vi "reset_TRIG2.vi"(8 "error in (no error)":errorcluster, 11 "VISA resource name":refnum<visa-resource-name>) -> (0 "error out":errorcluster, 3 "VISA resource name out":refnum<visa-resource-name>)   [LabVIEW 2011]
doc: "This vi resets TRIG2 (DG645) to its defaultsetup and then configures a default setup for the chirped pulse setup.\nThis includes activating the burst mode (3 bursts, 100us burst period), setting polarities as well as setting all delays and durations to 0."
uses:
  global.vi
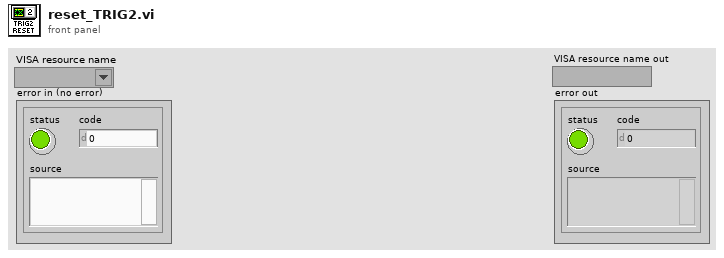
[diagram p1: front panel]
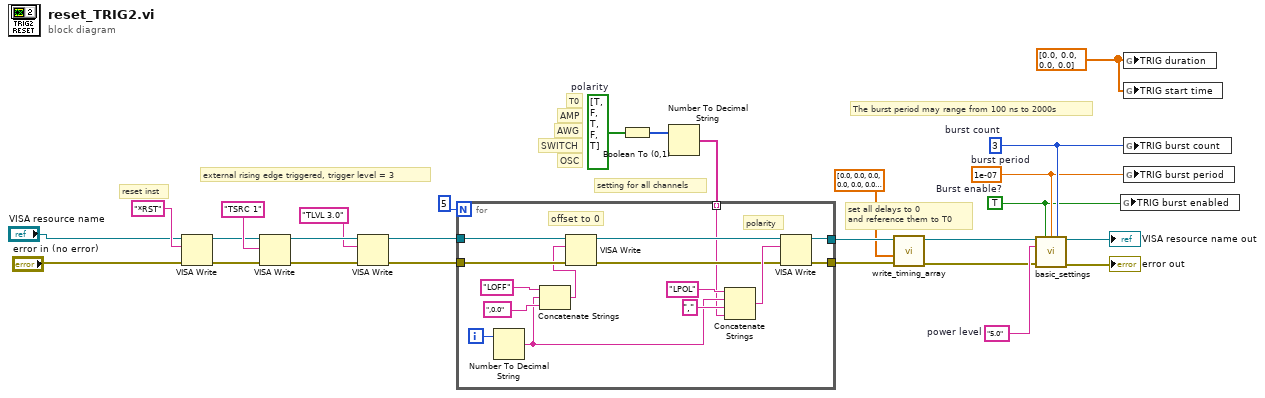
[diagram p0: block diagram]
diagram:
  w6 = bool[] [TRUE, FALSE, TRUE, FALSE, TRUE]  # polarity
  w9 = dbl[] [0.0, 0.0, 0.0, 0.0] ("duration")
  w16 = 3  # burst count
  w15 = 1e-07  # burst period
  w14 = TRUE  # Burst enable?
  w21 = "5.0"  # power level
  # "OSC"
  # "SWITCH"
  # "AWG"
  # "AMP"
  # "T0"
  # "The burst period may range from 100 ns to 2000s"
  # "set all delays to 0 \nand reference them to T0"
  # "reset inst"
  # "setting for all channels"
  # "external rising edge triggered, trigger level = 3"
  n1 = VISA Write(VISA resource name="VISA resource name", write buffer="*RST", error in (no error)="error in (no error)") -> (VISA resource name out=w23:refnum<visa-resource-name>, error out=w24:errorcluster)  [unwired: 1 out]
  n2 = VISA Write(VISA resource name=w23, write buffer="TSRC 1" ("Query 2"), error in (no error)=w24) -> (VISA resource name out=w3:refnum<visa-resource-name>, error out=w25:errorcluster)  [unwired: 1 out]
  n3 = VISA Write(VISA resource name=w3, write buffer="TLVL 3.0", error in (no error)=w25) -> (VISA resource name out=w2:refnum<visa-resource-name>, error out=w4:errorcluster)  [unwired: 1 out]
  n4 = Boolean To (0,1)(Boolean=w6) -> (0, 1=w7:i16[])
  n5 = Number To Decimal String(number=w7) -> (decimal integer string=w5:string[])  [unwired: 1 in]
  n6 = for {
    N: 5 -> [_]
    tunnel: w2 -> [w40]
    tunnel: [w31] -> w13
    tunnel: w4 -> [w39]
    tunnel: [w30] -> w12
    tunnel: w5 -> [w28] mode=indexing
    i -> [w38]
    # "polarity"
    # "offset to 0"
    n7 = Number To Decimal String(number=w38) -> (decimal integer string=w29:string)  [unwired: 1 in]
    n8 = Concatenate Strings("LOFF" ("Query 2"), w29, ",0.0" ("Query 2")) -> (w35:string)
    n9 = VISA Write(VISA resource name=w40, write buffer=w35, error in (no error)=w39) -> (VISA resource name out=w31:refnum<visa-resource-name>, error out=w30:errorcluster)  [unwired: 1 out]
    n10 = Concatenate Strings("LPOL" ("Query 2"), w29, "," ("string"), w28) -> (w33:string)
    n11 = VISA Write(VISA resource name=w31, write buffer=w33, error in (no error)=w30) -> ()  [unwired: 3 out]
  }
  n12 = call "write_timing_array.vi"("error in"=w12, "delay array"=dbl[] [0.0, 0.0, 0.0, 0.0, 0.0, 0.0, 0.0, 0.0] ("duration"), "VISA resource in"=w13) -> ("error out 2"=w10:errorcluster, "VISA resource out"=w11:refnum<visa-resource-name>)  [unwired: 3 in]
  n13 = call "basic_settings.vi"("VISA resource name"=w11, "Burst enable?"=w14, "burst period (s)"=w15, "burst count"=w16, "power level"=w21, "error in (no error)"=w10) -> ("VISA resource name out"=→"VISA resource name out":refnum<visa-resource-name>, "error out"=→"error out":errorcluster)  [unwired: 8 in]
  n14 = global write "global.vi" "TRIG burst enabled"(w14) -> ()
  n15 = global write "global.vi" "TRIG duration"(w9) -> ()
  n16 = global write "global.vi" "TRIG start time"(w9) -> ()
  n17 = global write "global.vi" "TRIG burst count"(w16) -> ()
  n18 = global write "global.vi" "TRIG burst period"(w15) -> ()
